vi "Close Connection.vi"(8 "error in (no error)":errorcluster, 11 "TCPConnection in":refnum<class "TCPConnection.lvclass">) -> (0 "error out":errorcluster, 3 "TCPConnection out":refnum<class "TCPConnection.lvclass">)   [LabVIEW 2013]
uses:
  TCPConnection.lvclass
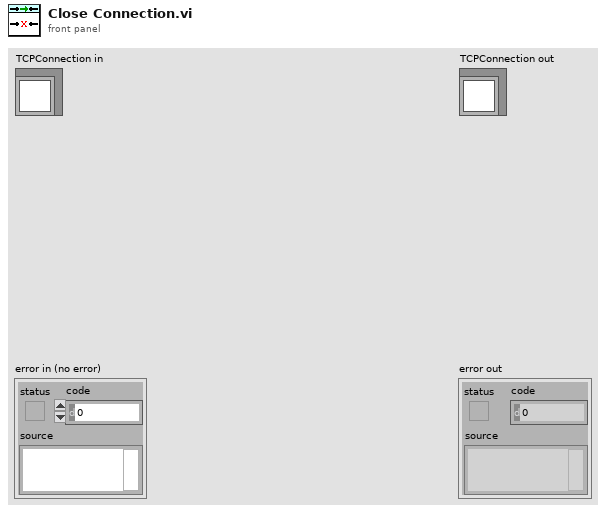
[diagram p1: front panel]
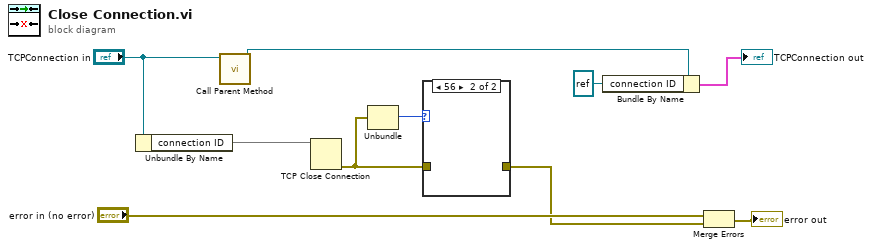
[diagram p0: block diagram]
diagram:
  n1 = Unbundle By Name("TCPConnection in") -> ("connection ID"=w6)
  n2 = call-parent "Call Parent Method"("Connection in"="TCPConnection in") -> ("Connection out"=w1:refnum<class "TCPConnection.lvclass">)  [unwired: 9 in, 1 out]
  n3 = TCP Close Connection(connection ID=w6) -> (error out=w3:errorcluster)  [unwired: 2 in, 1 out]
  n4 = Unbundle(w3) -> ("code"=w4:i32)  [unwired: 2 out]
  n5 = case shown="56" w4 {
    tunnel: w3 -> [w11 _]
    tunnel: [w11 _] -> w5
    frame Default {
    }
    frame 56 {
    }
  }
  n6 = Bundle By Name(cluster=w1, "connection ID"=refnum<k5> refnum) -> (→"TCPConnection out":cluster{})
  n7 = Merge Errors("error in (no error)", w5) -> (→"error out":errorcluster)
